vi "Scale Data 10x I16.vi"(3 "Data In":dbl format="%#_13g") -> (1 "16bit integer":i16)   [LabVIEW 2014]
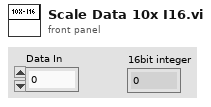
[diagram p1: front panel]
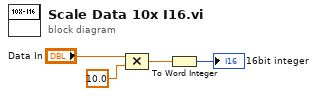
[diagram p0: block diagram]
diagram:
  n1 = Compound Arithmetic op=MULTIPLY("Data In", 10.0 ("value")) -> (w2:dbl)
  n2 = To Word Integer(number=w2) -> (16bit integer=→"16bit integer":i16)
